vi "Configure.vi"(8 "error in (no error)":errorcluster, 11 "DAQMH121119OrcaFlash in":refnum<class "DAQOrcaFlash.lvclass">) -> (0 "error out":errorcluster, 2 "cancelled?":bool, 3 "DAQMH121119OrcaFlash out":refnum<class "DAQOrcaFlash.lvclass">)   [LabVIEW 2012, in "DAQOrcaFlash.lvclass"]
doc: "The configure method configures the details for the RabbitMQ connection. \n\nIn the derived class, make a call to the parent for setting these parameters."
uses:
  DAQOrcaFlash.lvclass
  trigger_source.ctl
  read out direction.ctl
  sensor_mode.ctl
  trigger_mode.ctl
  output trigger type.ctl
  connector.ctl
  output trigger period.ctl
  trigger_polarity.ctl
  <vilib>/Utility/miscctls.llb/LVPointTypeDef.ctl
  DAQOrcaFlash.lvclass/DAQOrcaFlash.ctl
  <vilib>/Distrio/Murmex/Murmex/Murmex.lvclass
  output trigger source.ctl
panel:
  in  "Tab Control":T1(tab)=enum."Trigger"
  in  "Sensor mode":T2=12.0 items=["Normal"=1, "Light sheet"=12]
  in  "Read out direction":T3=1.0 items=["Top to Bottom"=1, "Bottom to Top"=2]
  in  "Trigger polarity":T4 items=["Negative"=1, "Positive"=2]
  in  "Output trigger period":T5=1e-05 min=5e-06 max=10 format="%#_6e"
  in  "Output trigger connector":T6
  in  "Output trigger type":T7=1.0 items=["Low"=1, "Global exposure"=2, "Programmable"=3, "Trigger ready"=4, "High"=5]
  in  "Trigger mode":T8=1.0 items=["Normal"=1, "Start"=6]
  in  "Trigger source":T9=2.0 items=["Internal"=1, "External"=2, "Software"=3]
  in  "Output trigger source":sgl(ring)=2.0 items=["READOUTEND"=2, "VSYNC"=3, "HSYNC"=4]
  in  "Output trigger polarity":T4 items=["Negative"=1, "Positive"=2]
  in  "relay start/stop to...":i32(listbox)
  in  "button:removeRelayTarget":bool
  in  "button:addRelayTarget":bool
  in  "relay target ID":string caption="target component ID"
  in  "storage directory":path=path "R:/test_hamamatsu"
  in  "maximum window size":dbl=1024.0 caption="px"
  in  "Autofocus component":string
  in  "final destination folder path (for conversion)":path
  in  "Tomo component":string
  in  "Stack component":string
  in  "auxiliary folders pahts (for conversion)":path[](array[path])
  in  "button:cancel":bool
  in  "button:ok":bool
  in  "button:configure_murmex":bool
  # "input Trigger"
  # "output trigger"
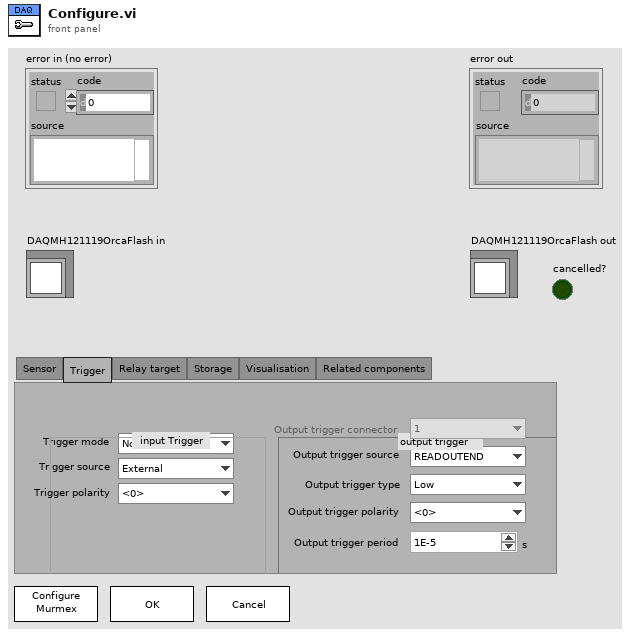
[diagram p1: front panel]
types:
  T1 = enum32{"Sensor", "Trigger", "Relay target", "Storage", "Visualisation", "Related components"}
  T2 = typedef "DAQOrcaFlash.lvclass/sensor_mode.ctl" = sgl
  T3 = typedef "DAQOrcaFlash.lvclass/read out direction.ctl" = sgl
  T4 = typedef "DAQOrcaFlash.lvclass/trigger_polarity.ctl" = sgl
  T5 = typedef "DAQOrcaFlash.lvclass/output trigger period.ctl" = sgl[unit]
  T6 = typedef "DAQOrcaFlash.lvclass/connector.ctl" = enum32{"1", "2", "3"}
  T7 = typedef "DAQOrcaFlash.lvclass/output trigger type.ctl" = sgl
  T8 = typedef "DAQOrcaFlash.lvclass/trigger_mode.ctl" = sgl
  T9 = typedef "DAQOrcaFlash.lvclass/trigger_source.ctl" = sgl
  T10 = enum32{"Sensor", "Trigger", "Relay target", "Storage"}
  T11 = typedef "LVPointTypeDef.ctl" = cluster{"Horizontal":i16, "Vertical":i16}
  T12 = typedef "DAQOrcaFlash.lvclass/output trigger source.ctl" = sgl
  T13 = enum8{"Enabled", "Disabled", "Disabled and Grayed Out"}
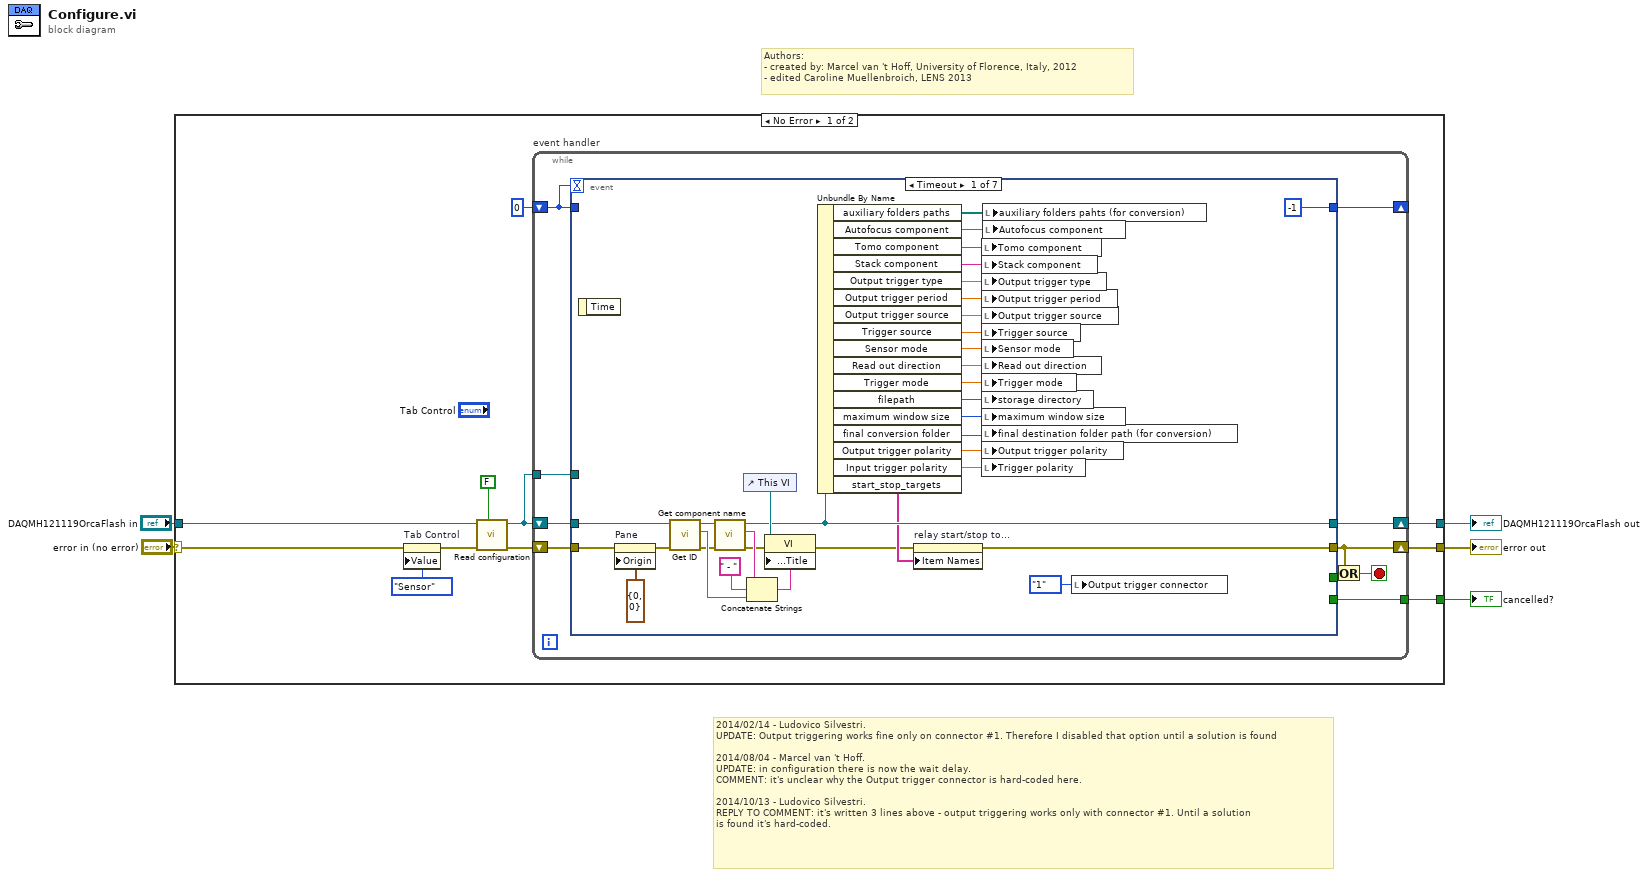
[diagram p0: block diagram]
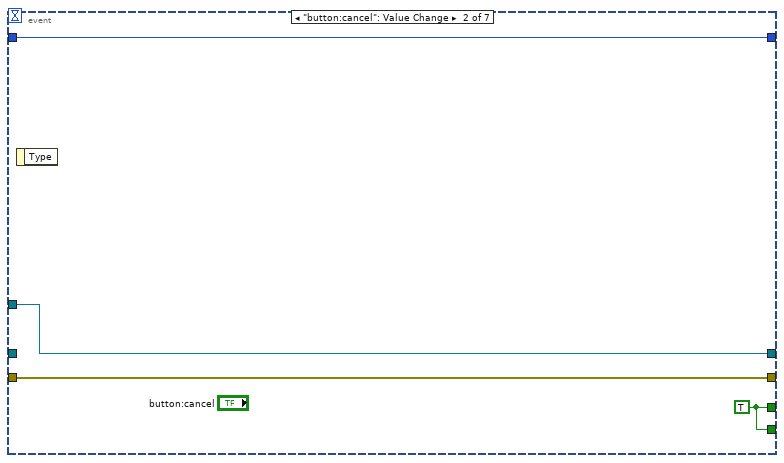
[diagram p2: hidden frame]
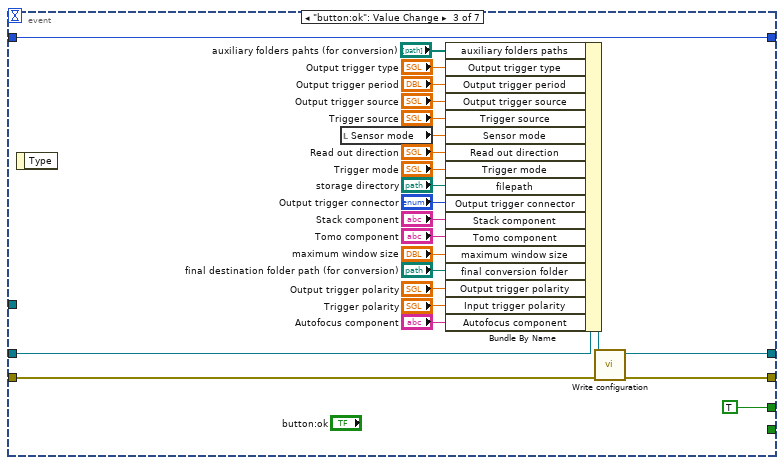
[diagram p3: hidden frame]
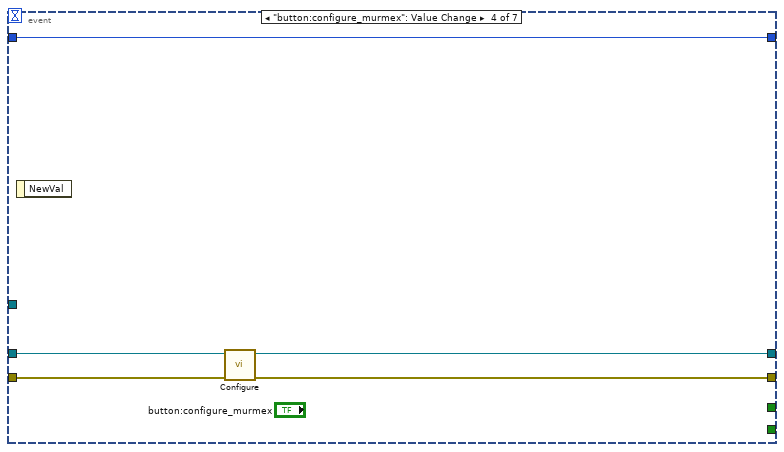
[diagram p4: hidden frame]
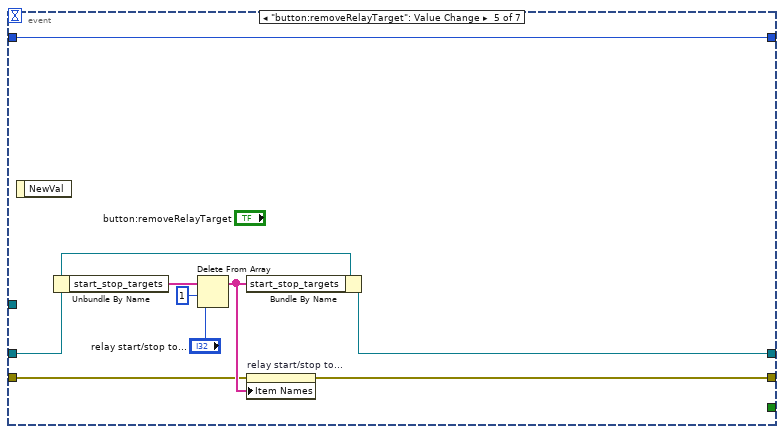
[diagram p5: hidden frame]
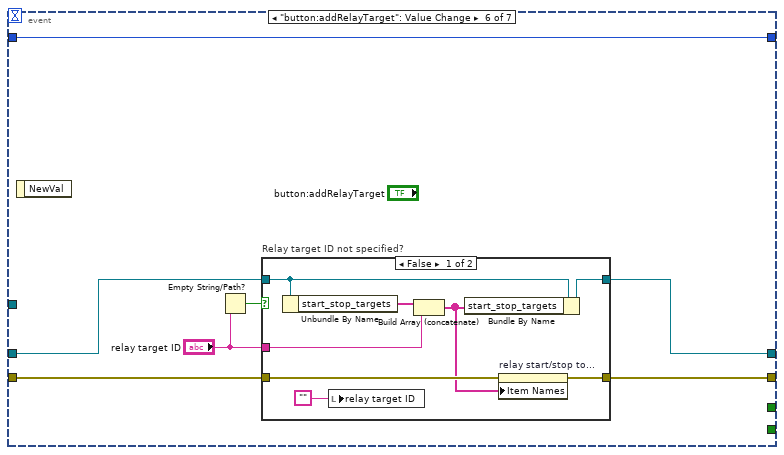
[diagram p6: hidden frame]
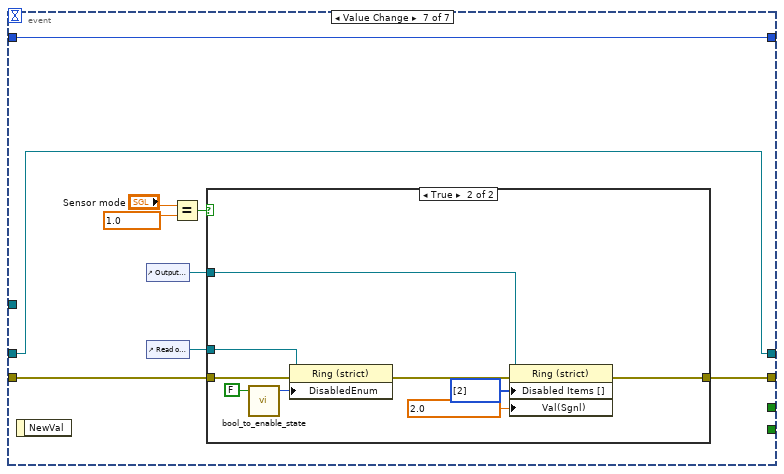
[diagram p8: hidden frame]
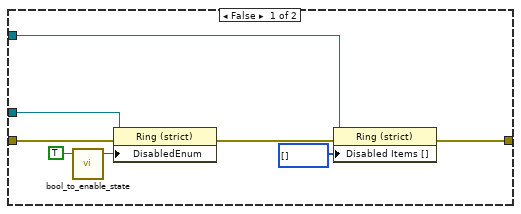
[diagram p9: hidden frame]
diagram:
  # "2014/02/14 - Ludovico Silvestri.\nUPDATE: Output triggering works fine only on connector #1. Therefore I disabled that option until a solution is found\n\n2014/08/04 - Marcel van 't Hoff.\nUPDATE: in configuration there is now the wait delay.\nCOMMENT: it's unclear why the Output trigger connector is hard-coded here.\n\n2014/10/13 - Ludovico Silvestri.\nREPLY TO COMMENT: it's written 3 lines above - output triggering works only with connector #1. Until a solution\nis found it's hard-coded."
  # "Authors: \n- created by: Marcel van 't Hoff, University of Florence, Italy, 2012\n- edited Caroline Muellenbroich, LENS 2013"
  n1 = case shown="No Error" "error in (no error)" {
    selector: "error in (no error)" -> [w7 w146]
    tunnel: [w16 w146] -> w5
    tunnel: [w15 w147] -> w1
    tunnel: [w13 _] -> w4
    tunnel: "DAQMH121119OrcaFlash in" -> [w10 w147]
    frame No Error {
      n2 = property on="Tab Control" class="TabCtl (strict)"(error in=w7, "Value"=T10."Sensor" ("Tab Control")) -> (error out=w6:errorcluster)  [unwired: 1 in, 1 out]
      n3 = call-dynamic "Read configuration.vi"("force loading?"=FALSE, "error in (no error)"=w6, "DAQMH121119OrcaFlash in"=w10) -> ("error out"=w11:errorcluster, "DAQMH121119OrcaFlash out"=w9:refnum<class "DAQOrcaFlash.lvclass">)  [unwired: 7 in]
      n4 = while "event handler" {
        shift-right: [w23] -> w16
        shift-left: w11 -> [w25]
        shift-right: [w26] -> w15
        shift-left: w9 -> [w24]
        shift-right: [w21] -> _
        shift-left: 0 -> [w20]
        tunnel: [w18] -> w13
        tunnel: w9 -> [w17]
        stop <- w22 stop-if-true
        n5 = event shown="[0] Timeout" {
          selector: _ -> [_ _ _ _ _ _ _]
          dyn-events: _ -> [_ _ _ _ _ _ _]
          timeout: w20 -> [_ _ _ _ _ _ _]
          tunnel: [w36 w64 w85 w93 w95 w104 w121] -> w23
          tunnel: [w39 w61 w84 w92 w99 w106 w120] -> w26
          tunnel: w25 -> [w57 w64 w88 w91 w96 w105 w124]
          tunnel: w24 -> [w60 _ w83 w90 w100 w107 w120]
          tunnel: [-1 w63 w87 w89 w94 w103 w128] -> w21
          tunnel: w20 -> [_ w63 w87 w89 w94 w103 w128]
          tunnel: [_ w62 TRUE _ _ _ _] -> w19
          tunnel: [_ w62 _ _ _ _ _] -> w18
          tunnel: w17 -> [_ w61 _ _ _ _ _]
          event Timeout {
            n6 = event-data() -> ()  [unwired: 1 in, 1 out]
            n7 = property on="Pane" class="Pane"(error in=w57, "Origin"=T11 {"Horizontal"=0, "Vertical"=0}) -> (error out=w52:errorcluster)  [unwired: 1 in, 1 out]
            n8 = call <vilib>:"Get ID.vi"("error in (no error)"=w52, "Murmex in"=w60) -> ("error out"=w51:errorcluster, "component id"=w54:string, "Murmex out"=w56:refnum<class "DAQOrcaFlash.lvclass">)  [unwired: 7 in]
            n9 = call <vilib>:"Get component name.vi"("error in (no error)"=w51, "Murmex in"=w56) -> ("error out"=w40:errorcluster, "component name"=w55:string, "Murmex out"=w39:refnum<class "DAQOrcaFlash.lvclass">)  [unwired: 7 in]
            n10 = control-ref of="This VI"() -> (w41:refnum<vi>)
            n11 = Concatenate Strings(w55, " - " ("string"), w54) -> (w42:string)
            n12 = property class="VI"(reference=w41, error in=w40, "Front Panel.Title"=w42) -> (error out=w37:errorcluster)  [unwired: 1 out]
            n13 = Unbundle By Name(w39) -> ("auxiliary folders paths"=w28:path[], "Autofocus component"=w27:string, "Tomo component"=w33:string, "Stack component"=w34:string, "Output trigger type"=w43:T7, "Output trigger period"=w44:sgl[unit], "Output trigger source"=w45:T12, "Trigger source"=w49:T9, "Sensor mode"=w48:T2, "Read out direction"=w47:T3, "Trigger mode"=w46:T8, "filepath"=w50:path, "maximum window size"=w32:i32, "final conversion folder"=w31:path, "Output trigger polarity"=w30:T4, "Input trigger polarity"=w29:T4, "start_stop_targets"=w38:string[])
            n14 = property on="relay start/stop to..." class="LstBox (strict)"(error in=w37, "Item Names"=w38) -> (error out=w36:errorcluster)  [unwired: 1 in, 1 out]
            n15 = local write "Tomo component"(w33) -> ()
            n16 = local write "Stack component"(w34) -> ()
            n17 = local write "Output trigger type"(w43) -> ()
            n18 = local write "Output trigger period"(w44) -> ()
            n19 = local write "Output trigger source"(w45) -> ()
            n20 = local write "Trigger source"(w49) -> ()
            n21 = local write "Sensor mode"(w48) -> ()
            n22 = local write "Read out direction"(w47) -> ()
            n23 = local write "Trigger mode"(w46) -> ()
            n24 = local write "storage directory"(w50) -> ()
            n25 = local write "maximum window size"(w32) -> ()
            n26 = local write "final destination folder path (for conversion)"(w31) -> ()
            n27 = local write "Output trigger polarity"(w30) -> ()
            n28 = local write "Trigger polarity"(w29) -> ()
            n29 = local write "auxiliary folders pahts (for conversion)"(w28) -> ()
            n30 = local write "Autofocus component"(w27) -> ()
            n31 = local write "Output trigger connector"(connector."1" ("configuration.Output trigger connector")) -> ()
          }
          event "button:cancel": Value Change {
            w62 = TRUE
            n32 = event-data() -> ()  [unwired: 1 in, 1 out]
          }
          event "button:ok": Value Change {
            n33 = event-data() -> ()  [unwired: 1 in, 1 out]
            n34 = local read "Sensor mode"() -> (w74:T2)
            n35 = Bundle By Name(cluster=w83, "auxiliary folders paths"="auxiliary folders pahts (for conversion)", "Output trigger type"="Output trigger type", "Output trigger period"="Output trigger period", "Output trigger source"="Output trigger source", "Trigger source"="Trigger source", "Sensor mode"=w74, "Read out direction"="Read out direction", "Trigger mode"="Trigger mode", "filepath"="storage directory", "Output trigger connector"="Output trigger connector", "Stack component"="Stack component", "Tomo component"="Tomo component", "maximum window size"="maximum window size", "final conversion folder"="final destination folder path (for conversion)", "Output trigger polarity"="Output trigger polarity", "Input trigger polarity"="Trigger polarity", "Autofocus component"="Autofocus component") -> (w82:refnum<class "DAQOrcaFlash.lvclass">)
            n36 = call-dynamic "Write configuration.vi"("error in (no error)"=w88, "DAQMH121119OrcaFlash in"=w82) -> ("error out"=w85:errorcluster, "DAQMH121119OrcaFlash out"=w84:refnum<class "DAQOrcaFlash.lvclass">)  [unwired: 8 in]
          }
          event "button:configure_murmex": Value Change {
            n37 = event-data() -> ()  [unwired: 1 in, 1 out]
            n38 = call-parent "Configure.vi"("error in (no error)"=w91, "Murmex in"=w90) -> ("error out"=w93:errorcluster, "Murmex out"=w92:refnum<class "DAQOrcaFlash.lvclass">)  [unwired: 7 in, 1 out]
          }
          event "button:removeRelayTarget": Value Change {
            n39 = event-data() -> ()  [unwired: 1 in, 1 out]
            n40 = Unbundle By Name(w100) -> ("start_stop_targets"=w102:string[])
            n41 = Delete From Array(array=w102, length=1, index="relay start/stop to...") -> (array with subset deleted=w97:string[])  [unwired: 1 out]
            n42 = Bundle By Name(cluster=w100, "start_stop_targets"=w97) -> (w99:refnum<class "DAQOrcaFlash.lvclass">)
            n43 = property on="relay start/stop to..." class="LstBox (strict)"(error in=w96, "Item Names"=w97) -> (error out=w95:errorcluster)  [unwired: 1 in, 1 out]
          }
          event "button:addRelayTarget": Value Change {
            n44 = event-data() -> ()  [unwired: 1 in, 1 out]
            n45 = Empty String/Path?(string/path="relay target ID") -> (empty?=w109:bool)
            n46 = case "Relay target ID not specified?" shown="False" w109 {
              tunnel: w107 -> [w116 w119]
              tunnel: [w115 w119] -> w106
              tunnel: "relay target ID" -> [w114 _]
              tunnel: w105 -> [w112 w118]
              tunnel: [w111 w118] -> w104
              frame False {
                n47 = Unbundle By Name(w116) -> ("start_stop_targets"=w117:string[])
                n48 = local write "relay target ID"("") -> ()
                n49 = Build Array (concatenate)(w117, w114) -> (w110:string[])
                n50 = Bundle By Name(cluster=w116, "start_stop_targets"=w110) -> (w115:refnum<class "DAQOrcaFlash.lvclass">)
                n51 = property on="relay start/stop to..." class="LstBox (strict)"(error in=w112, "Item Names"=w110) -> (error out=w111:errorcluster)  [unwired: 1 in, 1 out]
              }
              frame True {
              }
            }
          }
          event Value Change {
            w126 = T2 1.0 items=["Normal"=1.0, "Light sheet"=12.0] ("y")
            n52 = event-data() -> ()  [unwired: 1 in, 1 out]
            n53 = control-ref of="Output trigger source"() -> (w122:refnum<vi>)
            n54 = control-ref of="Read out direction"() -> (w123:refnum<vi>)
            n55 = Equal?(x="Sensor mode", y=w126) -> (x = y?=w125:bool)
            n56 = case shown="True" w125 {
              tunnel: w124 -> [w133 w144]
              tunnel: w123 -> [w132 w145]
              tunnel: w122 -> [w131 w141]
              tunnel: [w129 w139] -> w121
              frame False {
                n57 = call "bool_to_enable_state.vi"("boolean in"=TRUE) -> ("enabled status out"=w136:T13)  [unwired: 4 in]
                n58 = property class="Ring (strict)"(reference=w132, error in=w133, "DisabledEnum"=w136) -> (error out=w134:errorcluster)  [unwired: 1 out]
                n59 = property class="Ring (strict)"(reference=w131, error in=w134, "Disabled Items []"=i32[] []) -> (error out=w129:errorcluster)  [unwired: 1 out]
              }
              frame True {
                w137 = T12 2.0 items=["READOUTEND"=2.0, "VSYNC"=3.0, "HSYNC"=4.0] ("Value (Signaling)")
                n60 = call "bool_to_enable_state.vi"("boolean in"=FALSE) -> ("enabled status out"=w143:T13)  [unwired: 4 in]
                n61 = property class="Ring (strict)"(reference=w145, error in=w144, "DisabledEnum"=w143) -> (error out=w140:errorcluster)  [unwired: 1 out]
                n62 = property class="Ring (strict)"(reference=w141, error in=w140, "Disabled Items []"=i32[] [2], "Val(Sgnl)"=w137) -> (error out=w139:errorcluster)  [unwired: 1 out]
              }
            }
          }
        }
        n63 = Or(x=w23, y=w19) -> (x .or. y?=w22:bool)
      }
    }
    frame Error {
    }
  }
  "error out" <- w5
  "DAQMH121119OrcaFlash out" <- w1
  "cancelled?" <- w4
